vi "Read Humidity.vi"(8 "error in (no error)":errorcluster, 11 "wait for target (50)":u32=50) -> (0 "error out":errorcluster, 2 "temperature (°C)":u8, 3 "humidity (%)":u8)   [LabVIEW 2015]
doc: "A DIO 0"
uses:
  <vilib>/rvi/interface/nirviOpenFPGA/nirviOpenFPGA.xnode
  <vilib>/rvi/interface/nirviReadWriteControl/nirviReadWriteControl.xnode
  NiFpgaLv.dll
  <vilib>/Utility/error.llb/Error Cluster From Error Code.vi
  <vilib>/rvi/interface/Simulation/niFpgaSimulationCallBeginRW.vi
  <vilib>/rvi/errors/niLvFpgaAdjustHostInterfaceError.vi
  <vilib>/rvi/interface/nirviCloseFPGA/nirviCloseFPGA.xnode
  <vilib>/FPGAPlugInAG/Dynamic/niLvFpga_Close_Dynamic.vi
  FPGA Bitfiles/IoTFoundationDEM_FPGATarget_DHT11(FPGA)_nBL-L-qrK6U.lvbitx
  DHT11 Library/DHT11 (FPGA).vi
  <vilib>/FPGAPlugInAG/myRIO-1900/niLvFpga_Open_myRIO-1900.vi
  <vilib>/rvi/interface/common/dynamic/niFpgaDynamicAddResources.vi
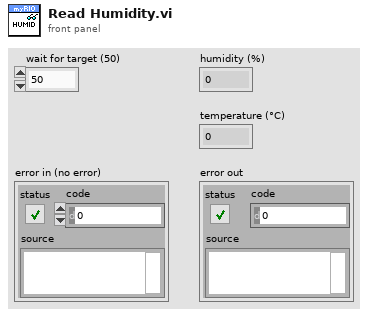
[diagram p1: front panel]
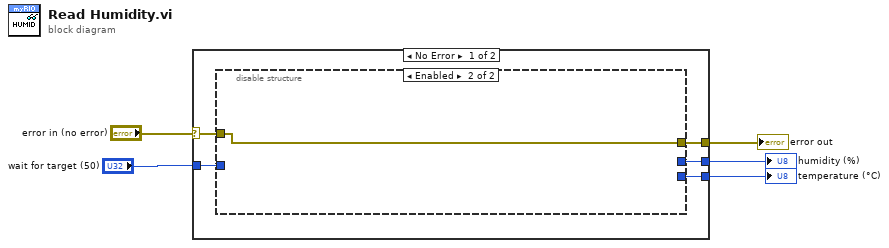
[diagram p0: block diagram]
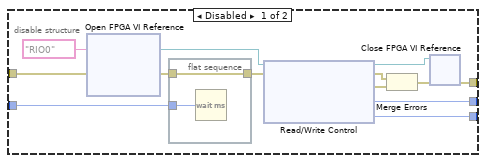
[diagram p2: hidden frame]
diagram:
  n1 = case shown="No Error" "error in (no error)" {
    selector: "error in (no error)" -> [w8 w27]
    tunnel: "wait for target (50)" -> [w10 _]
    tunnel: [w9 w27] -> w2
    tunnel: [w7 _] -> w4
    tunnel: [w6 _] -> w5
    frame No Error {
      n2 = disable-structure shown="Enabled" {
        disable-tunnel: w10 -> [w18 _]
        disable-tunnel: [w14 w26] -> w9
        disable-tunnel: w8 -> [w13 w26]
        disable-tunnel: [w12 _] -> w7
        disable-tunnel: [w11 _] -> w6
        frame Disabled {
          n3 = xnode "Open FPGA VI Reference"("error in"=w13, "resource name"=tag "RIO0") -> ("FPGA VI Reference Out"=w19:refnum<k20>, "error out"=w21:errorcluster)
          n4 = flat-sequence {
            tunnel: [w25] -> w20
            tunnel: w21 -> [w25]
            tunnel: w18 -> [w24]
            frame #0 {
              n5 = Wait (ms)(milliseconds to wait=w24) -> ()  [unwired: 1 out]
            }
          }
          n6 = xnode "Read/Write Control"("FPGA VI Reference In"=w19, "error in"=w20) -> ("FPGA VI Reference Out"=w22:refnum<k20>, "error out"=w17:errorcluster, "error out"=w16:errorcluster, "Humidity (%)"=w12:u8, "Temperature (°C)"=w11:u8)
          n7 = Merge Errors(w17, w16) -> (w15:errorcluster)
          n8 = xnode "Close FPGA VI Reference"("FPGA VI Reference In"=w22, "error in"=w15) -> ("error out"=w14:errorcluster)
        }
        frame Enabled {
        }
      }
    }
    frame Error {
    }
  }
  "temperature (°C)" <- w5
  "humidity (%)" <- w4
  "error out" <- w2
